vi "TSCAN Init.vi"(0 "路径输入":path, 11 "错误输入（无错误）":errorcluster) -> (4 "路径输出":path, 15 "错误输出":errorcluster)   [LabVIEW 2013]
panel:
  out "Init_TS_API_Successfully":bool
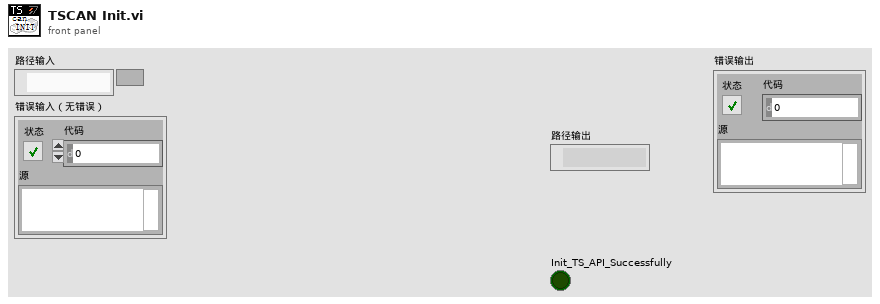
[diagram p1: front panel]
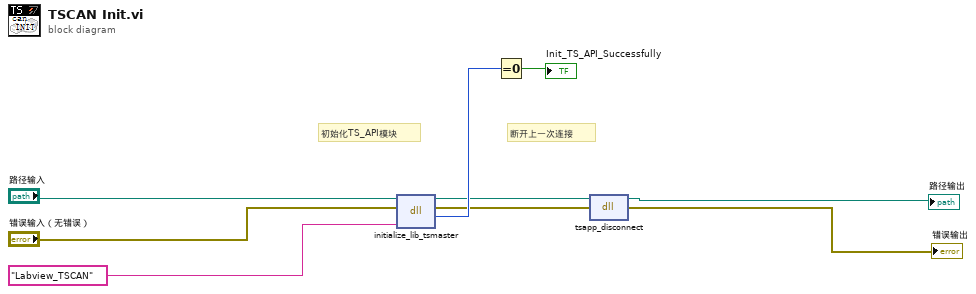
[diagram p0: block diagram]
diagram:
  # "断开上一次连接"
  # "初始化TS_API模块"
  n1 = dll-call lib="PTH1Habs CUsers\nAdministratorDesktopTS_Can通讯PathTSMaster.dll" fn="initialize_lib_tsmaster"(path in="路径输入", error in="错误输入（无错误）", "AppName"="Labview_TSCAN") -> (path out=w6:path, error out=w5:errorcluster, "Initialize_lib_tsmaster"=w8:i32)  [unwired: 2 in]
  n2 = Equal To 0?(x=w8) -> (x = 0?=→"Init_TS_API_Successfully":bool)
  n3 = dll-call lib="PTH1Zabs CUsers\nAdministratorDesktopLB2018TS_CAN通讯 文件夹PathTSMaster.dll" fn="tsapp_disconnect"(path in=w6, error in=w5) -> (path out=→"路径输出":path, error out=→"错误输出":errorcluster)  [unwired: 2 in]
